vi "EVENTbench.vi"() -> ()   [LabVIEW 2017]
panel:
  in  "testButton":bool=TRUE
  out "testlamp":bool=TRUE
  in  "Lemon squeezy":bool=TRUE
  out "String":string
  in  "Easy peasy":bool=TRUE
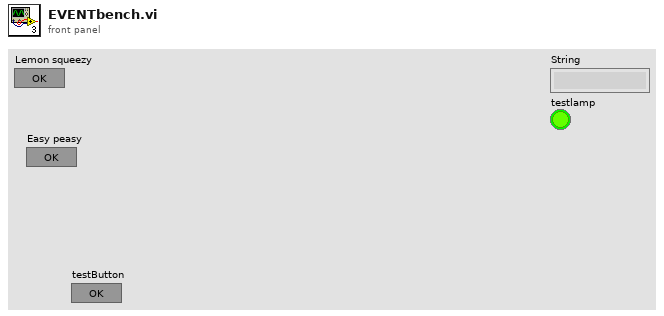
[diagram p1: front panel]
types:
  T1 = cluster{"str":string, "ctlref":refnum<vi>, "newStatus":bool}
  T2 = cluster{string, "chgStatusLED":refnum<user-event>}
  T3 = cluster{string, "chgStatusLED":refnum<user-event>}[]
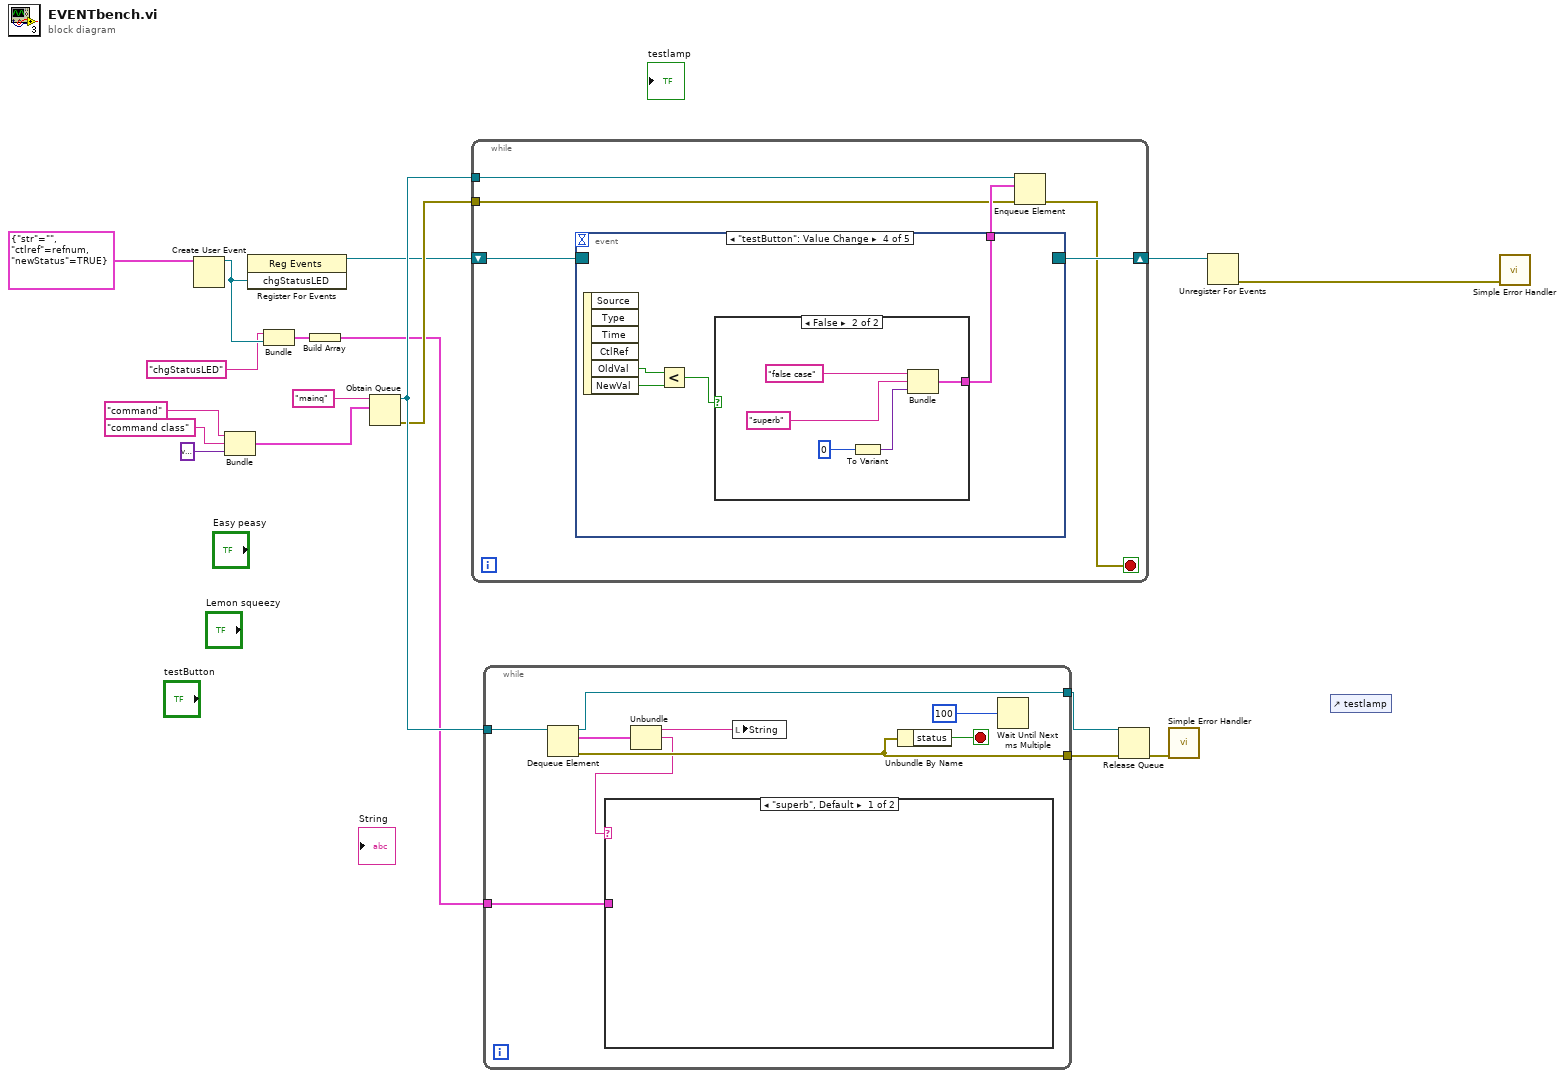
[diagram p0: block diagram]
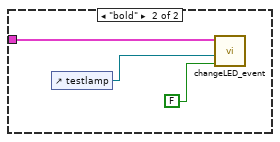
[diagram p2: hidden frame]
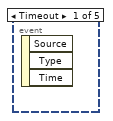
[diagram p3: hidden frame]
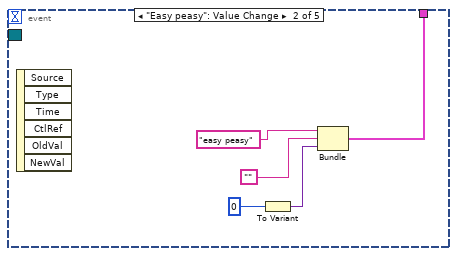
[diagram p4: hidden frame]
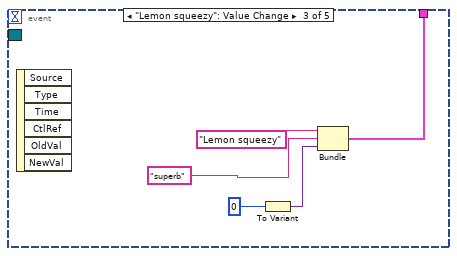
[diagram p5: hidden frame]
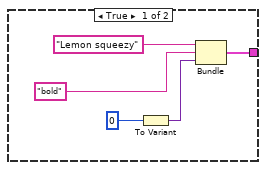
[diagram p6: hidden frame]
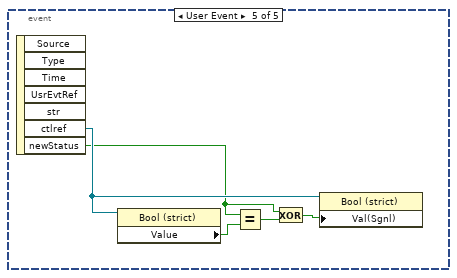
[diagram p7: hidden frame]
diagram:
  n1 = Create User Event(user event datatype=T1 {"str"="", "ctlref"=refnum, "newStatus"=TRUE} ("chgStatusLED")) -> (user event=w5:refnum<user-event>)  [unwired: 1 in, 1 out]
  n2 = Bundle("command", "command class", variant) -> (w14:cluster{string, string, variant})  [unwired: 1 in]
  n3 = register-events(w5) -> (reference out=w6:refnum<event-registration>)  [unwired: 2 in, 1 out]
  n4 = Bundle("chgStatusLED", "chgStatusLED"=w5) -> (w3:T2)  [unwired: 1 in]
  n5 = Build Array(w3) -> (w2:T3)
  n6 = Obtain Queue(name (unnamed)="mainq", element data type=w14) -> (queue out=w13:refnum<queue>, error out=w8:errorcluster)  [unwired: 3 in, 1 out]
  n7 = while {
    tunnel: w13 -> [w24]
    shift-right: [w22] -> w10
    shift-left: w6 -> [w21]
    tunnel: w8 -> [w20]
    stop <- w19 stop-if-true
    n8 = event shown="[3] \"testButton\": Value Change" {
      selector: w21 -> [_ _ _ _ _]
      dyn-events: [_ _ _ _ _] -> w22
      timeout: _ -> [_ _ _ _ _]
      tunnel: [_ w25 w31 w38 _] -> w23
      event Timeout {
        n9 = event-data() -> ()  [unwired: 1 in, 3 out]
      }
      event "Easy peasy": Value Change {
        n10 = event-data() -> ()  [unwired: 1 in, 6 out]
        n11 = To Variant(anything=0) -> (Variant=w27:variant)
        n12 = Bundle("easy peasy", "", "Variant"=w27) -> (w25:cluster{string, string, "Variant":variant})  [unwired: 1 in]
      }
      event "Lemon squeezy": Value Change {
        n13 = event-data() -> ()  [unwired: 1 in, 6 out]
        n14 = To Variant(anything=0) -> (Variant=w33:variant)
        n15 = Bundle("Lemon squeezy", "superb", "Variant"=w33) -> (w31:cluster{string, string, "Variant":variant})  [unwired: 1 in]
      }
      event "testButton": Value Change {
        n16 = event-data() -> ("OldVal"=w36:bool, "NewVal"=w37:bool)  [unwired: 1 in, 4 out]
        n17 = Less?(x=w36, y=w37) -> (x < y?=w35:bool)
        n18 = case shown="False" w35 {
          tunnel: [w39 w44] -> w38
          frame True {
            n19 = To Variant(anything=0) -> (Variant=w42:variant)
            n20 = Bundle("Lemon squeezy", "bold", "Variant"=w42) -> (w39:cluster{string, string, "Variant":variant})  [unwired: 1 in]
          }
          frame False {
            n21 = To Variant(anything=0) -> (Variant=w47:variant)
            n22 = Bundle("false case", "superb", "Variant"=w47) -> (w44:cluster{string, string, "Variant":variant})  [unwired: 1 in]
          }
        }
      }
      event User Event {
        n23 = event-data() -> ("ctlref"=w53:refnum<vi>, "newStatus"=w49:bool)  [unwired: 1 in, 5 out]
        n24 = property on="Property Node" class="Bool (strict)"(reference=w53) -> ("Value"=w52:bool)  [unwired: 1 in, 2 out]
        n25 = Equal?(x=w49, y=w52) -> (x = y?=w51:bool)
        n26 = Exclusive Or(1:w51, 2:w49) -> (0:w50:bool)
        n27 = property on="Property Node" class="Bool (strict)"(reference=w53, "Val(Sgnl)"=w50) -> ()  [unwired: 1 in, 2 out]
      }
    }
    n28 = Enqueue Element(queue=w24, element=w23, error in (no error)=w20) -> (error out=w19:errorcluster)  [unwired: 1 in, 2 out]
  }
  n29 = while {
    tunnel: w13 -> [w61]
    tunnel: [w59] -> w11
    tunnel: [w56] -> w9
    tunnel: w2 -> [w54]
    stop <- w58 stop-if-true
    n30 = Dequeue Element(queue=w61) -> (queue out=w56:refnum<queue>, element=w60:cluster{string, string, variant}, error out=w59:errorcluster)  [unwired: 2 in, 1 out]
    n31 = Unbundle(w60) -> (w57:string, w55:string)  [unwired: 1 out]
    n32 = case shown="\"superb\", Default" w55 {
      tunnel: w54 -> [_ w65]
      frame "superb", Default {
      }
      frame "bold" {
        n33 = control-ref of="testlamp"() -> (w64:refnum<vi>)
        n34 = call "changeLED_event.vi"("Array"=w65, "ctlref"=w64, "newStatus"=FALSE) -> ()  [unwired: 7 in, 1 out]
      }
    }
    n35 = local write "String"(w57) -> ()
    n36 = Unbundle By Name(w59) -> ("status"=w58:bool)
    n37 = Wait Until Next ms Multiple(millisecond multiple=100) -> ()  [unwired: 1 out]
  }
  n38 = Release Queue(queue=w9, error in (no error)=w11) -> (error out=w12:errorcluster)  [unwired: 3 out]
  n39 = call <vilib>:"Simple Error Handler.vi"("error in (no error)"=w12) -> ()  [unwired: 1 in, 8 out]
  n40 = Unregister For Events(event registration refnum=w10) -> (error out=w1:errorcluster)  [unwired: 1 in]
  n41 = control-ref of="testlamp"() -> ()  [unwired: 1 out]
  n42 = call <vilib>:"Simple Error Handler.vi"("error in (no error)"=w1) -> ()  [unwired: 1 in, 8 out]
